vi "process_frame_text.vi"(11 "字符串":string) -> (3 "result string":string)   [LabVIEW 2020]
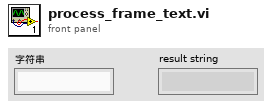
[diagram p1: front panel]
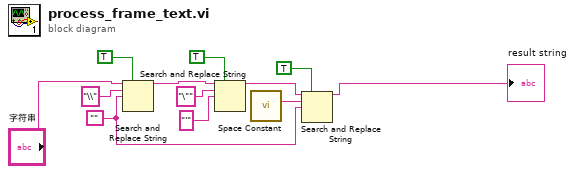
[diagram p0: block diagram]
diagram:
  w10 = ""
  n1 = Search and Replace String(replace all?=TRUE ("替换全部？(F)"), input string="字符串", search string="\\" ("搜索字符串"), replace string=w10) -> (result string=w3:string)  [unwired: 4 in, 3 out]
  n2 = Search and Replace String(replace all?=TRUE ("替换全部？(F)"), input string=w3, search string="\"" ("搜索字符串"), replace string="'" ("替换字符串(\"\")")) -> (result string=w9:string)  [unwired: 4 in, 3 out]
  n3 = call <vilib>:"Space Constant.vi"() -> ("String"=w11:string)
  n4 = Search and Replace String(replace all?=TRUE ("替换全部？(F)"), input string=w9, search string=w11, replace string=w10) -> (result string=→"result string":string)  [unwired: 4 in, 3 out]
